vi "manualTestWasRun.vi"() -> ()   [LabVIEW 2013]
uses:
  WasRun/WasRun.lvclass
panel:
  out "visual OK indicator":bool[](array[boolean])
  out "error out":errorcluster
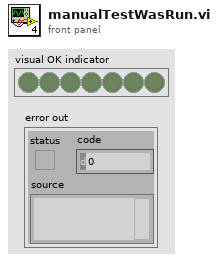
[diagram p1: front panel]
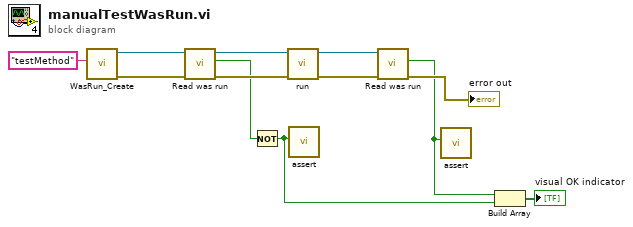
[diagram p0: block diagram]
diagram:
  n1 = call "WasRun_Create.vi"("Name"="testMethod") -> ("error out"=w10:errorcluster, "WasRun out"=w11:refnum<class "WasRun.lvclass">)  [unwired: 9 in]
  n2 = call-dynamic "Read was run.vi"("error in (no error)"=w10, "WasRun in"=w11) -> ("error out"=w6:errorcluster, "was run"=w3:bool, "WasRun out"=w8:refnum<class "WasRun.lvclass">)  [unwired: 7 in]
  n3 = Not(x=w3) -> (.not. x?=w1:bool)
  n4 = call "run.vi"("error in (no error)"=w6, "WasRun in"=w8) -> ("error out"=w5:errorcluster, "WasRun out"=w7:refnum<class "WasRun.lvclass">)  [unwired: 8 in]
  n5 = call "assert.vi"("mustBeTrue"=w1) -> ()  [unwired: 11 in]
  n6 = call-dynamic "Read was run.vi"("error in (no error)"=w5, "WasRun in"=w7) -> ("error out"=→"error out":errorcluster, "was run"=w4:bool)  [unwired: 7 in, 1 out]
  n7 = call "assert.vi"("mustBeTrue"=w4) -> ()  [unwired: 11 in]
  n8 = Build Array(w4, w1) -> (→"visual OK indicator":bool[])
